vi "Teleop.vi"(10 "Match Info":T1={"Autonomous Elapsed Seconds"=0.0, "TeleOp Elapsed Seconds"=0.0, "Disabled Elapsed Seconds"=0.0, "Visited Autonomous"=FALSE, "Visited TeleOp"=FALSE, "Visited Disabled"=FALSE, "Autonomous Settings"={"Autonomous Style"=enum."Independent", "VI Refnum"=refnum}}, 11 "Call Context":T2) -> ()   [LabVIEW 2014]
doc: "This VI is called for each TeleOp packet received from the DS where the robot is not disabled. It is often used to read from the joysticks and update I/O or to update setpoints for timed control loops. It should complete and return within 20 milliseconds or it may miss DS packets."
uses:
  <vilib>/Rock Robotics/WPI/DriverStation/WPI_DriverStationDerivedRobotMode.ctl
  <vilib>/Rock Robotics/WPI/DriverStation/WPI_DriverStationMatch Info.ctl
  <vilib>/Rock Robotics/WPI/RobotDrive/WPI_RobotDriveGetSetRefNum.vi
  <vilib>/Rock Robotics/WPI/Joystick/WPI_JoystickGetSetRefNum.vi
  <vilib>/Rock Robotics/Network Tables/SD Write Boolean Array.vi
  <vilib>/Rock Robotics/Network Tables/SD Write Numeric Array.vi
  Robot Global Data.vi
  <vilib>/Rock Robotics/Network Tables/SD Read Boolean.vi
  <vilib>/Rock Robotics/Network Tables/SD Read Number.vi
panel:
  out "Sample Slider 0":dbl(slide) scale=0.0..5.0
  out "Sample Boolean 1":bool
  out "Sample Boolean 0":bool
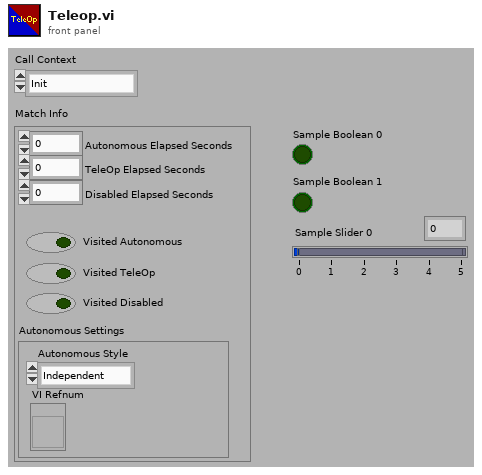
[diagram p1: front panel]
types:
  T1 = typedef "WPI_DriverStationMatch Info.ctl" = cluster{"Autonomous Elapsed Seconds":dbl, "TeleOp Elapsed Seconds":dbl, "Disabled Elapsed Seconds":dbl, "Visited Autonomous":bool, "Visited TeleOp":bool, "Visited Disabled":bool, "Autonomous Settings":cluster{"Autonomous Style":enum16{"Iterative", "Independent"}, "VI Refnum":refnum<vi>}}
  T2 = typedef "WPI_DriverStationDerivedRobotMode.ctl" = enum16{"Init", "Execute", "Stop"}
  T3 = typedef "WPI_RobotDriveDevRef.ctl" = cluster{"DevStatus":errorcluster, "Motors[]":T4[], "Square Inputs":bool, "Max Output":dbl}
  T4 = typedef "WPI_MotorControlDeviceRef.ctl" = cluster{"DeviceStatus":errorcluster, "Type":T5, "PWM":cluster{"Controller":T6, "PWM Channel":T7, "DeadBand":T8}, "CAN":cluster{"Device Number":u8, "Control Mode":T9, "Semaphore":T10, "Max Vout":dbl, "TalonSRX Control Mode":T11}, "Invert":bool, "TransformRef":T12, "InvTransformRef":T12}
  T5 = typedef "WPI_MotorControlType.ctl" = enum16{"PWM", "CAN", "CANTalonSRX"}
  T6 = typedef "FPGA_TypedefDigitalModule.ctl" = enum16{"Controller 1"}
  T7 = typedef "FPGA_DIOPWMChannel.ctl" = enum8{"PWM 0", "PWM 1", "PWM 2", "PWM 3", "PWM 4", "PWM 5", "PWM 6", "PWM 7", "PWM 8", "PWM 9", "PWM MXP 0", "PWM MXP 1", "PWM MXP 2", "PWM MXP 3", "PWM MXP 4", "PWM MXP 5", "PWM MXP 6", "PWM MXP 7", "PWM MXP 8", "PWM MXP 9", "Invalid"}
  T8 = typedef "WPI_PWMDeadband.ctl" = cluster{"Name":string, "maxPositivePwm":i32, "minPositivePwm":i32, "centerPwm":i32, "maxNegativePwm":i32, "minNegativePwm":i32, "angularRange":u16}
  T9 = typedef "WPI_CANJaguar_ControlMode.ctl" = enum8{"Percent VBus", "Current", "Speed", "Position", "Voltage"}
  T10 = typedef "Semaphore RefNum" = refnum<k1>
  T11 = typedef "WPI_CANTalonSRX_APIControlMode.ctl" = enum8{"Percent VBus", "Speed", "Position", "Slave", "Unchanged / Invalid"}
  T12 = typedef "WPI_PWMTransform_ConPane.ctl" = refnum<vi>
  T13 = typedef "WPI_JoystickDevRef.ctl" = cluster{"Device":T14}
  T14 = typedef "WPI_JoystickDeviceEnum.ctl" = enum16{"USB 0", "USB 1", "USB 2", "USB 3", "USB 4", "USB 5"}
  T15 = cluster{"Buttons[0]":bool, "Buttons[1]":bool, "Buttons[2]":bool, "Buttons[3]":bool, "Buttons[4]":bool, "Buttons[5]":bool, "Buttons[6]":bool, "Buttons[7]":bool, "Buttons[8]":bool}
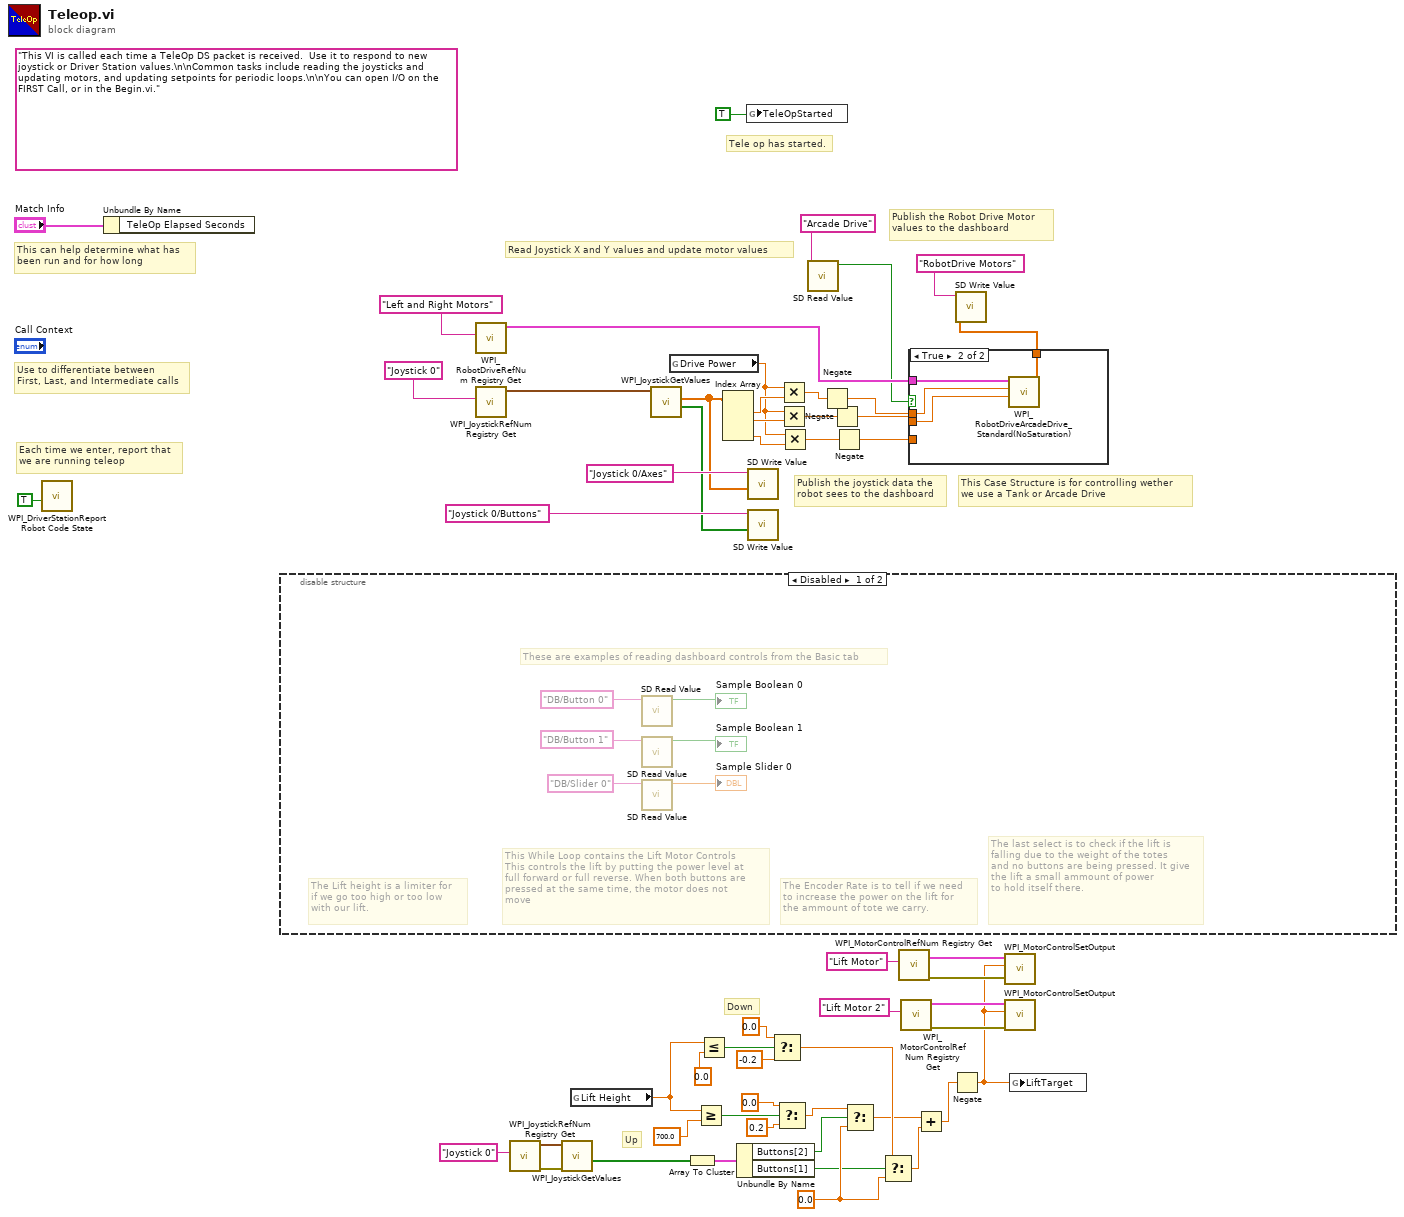
[diagram p0: block diagram]
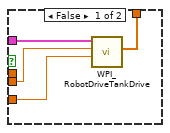
[diagram p3: hidden frame]
diagram:
  w20 = 0.0
  (unwired) "This VI is called each time a TeleOp DS packet is received.  Use it to respond to new joystick or Driver Station values.\n\nCommon tasks include reading the joysticks and updating motors, and updating setpoints for periodic loops.\n\nYou can open I/O on the FIRST Call, or in the Begin.vi."
  # "Read Joystick X and Y values and update motor values"
  # "Up"
  # "Down"
  # "Tele op has started."
  # "This Case Structure is for controlling wether\nwe use a Tank or Arcade Drive"
  # "Publish the Robot Drive Motor\nvalues to the dashboard"
  # "Publish the joystick data the\nrobot sees to the dashboard"
  # "Each time we enter, report that\nwe are running teleop"
  # "Use to differentiate between\nFirst, Last, and Intermediate calls"
  # "This can help determine what has\nbeen run and for how long"
  n1 = call <vilib>:"WPI_DriverStationReport Robot Code State.vi"("TeleOp"=TRUE ("Autonomous")) -> ()  [unwired: 10 in, 1 out]
  n2 = Unbundle By Name("Match Info") -> ()  [unwired: 1 out]
  n3 = disable-structure shown="Disabled" {
    frame Disabled {
      # "The last select is to check if the lift is falling due to the weight of the totes\nand no buttons are being pressed. It give the lift a small ammount of power\nto hold itself there."
      # "The Encoder Rate is to tell if we need\nto increase the power on the lift for\nthe ammount of tote we carry."
      # "The Lift height is a limiter for \nif we go too high or too low\nwith our lift."
      # "This While Loop contains the Lift Motor Controls\nThis controls the lift by putting the power level at\nfull forward or full reverse. When both buttons are\npressed at the same time, the motor does not\nmove"
      # "These are examples of reading dashboard controls from the Basic tab"
      n4 = call-poly <vilib>:"SD Read Value.vi"("Name"="DB/Button 0" ("refnum name")) -> ("Boolean"=→"Sample Boolean 0":bool)  [unwired: 8 in, 2 out]
      n5 = call-poly <vilib>:"SD Read Value.vi"("Name"="DB/Button 1" ("refnum name")) -> ("Boolean"=→"Sample Boolean 1":bool)  [unwired: 8 in, 2 out]
      n6 = call-poly <vilib>:"SD Read Value.vi"("Name"="DB/Slider 0" ("refnum name")) -> ("Numeric"=→"Sample Slider 0":dbl)  [unwired: 8 in, 2 out]
    }
    frame Enabled {
    }
  }
  n7 = call <vilib>:"WPI_RobotDriveRefNum Registry Get.vi"("refnum name"="Left and Right Motors") -> ("RobotDriveDevRef"=w38:T3)  [unwired: 1 in, 9 out]
  n8 = call <vilib>:"WPI_JoystickRefNum Registry Get.vi"("refnum name"="Joystick 0") -> ("JoystickDevRef"=w51:T13)  [unwired: 1 in, 9 out]
  n9 = call <vilib>:"WPI_JoystickRefNum Registry Get.vi"("refnum name"="Joystick 0") -> ("error out"=w29:errorcluster, "JoystickDevRef"=w30:T13)  [unwired: 9 in]
  n10 = call <vilib>:"WPI_JoystickGetValues.vi"("error in (no error)"=w29, "JoystickDevRef"=w30) -> ("Buttons"=w21:bool[])  [unwired: 5 in, 4 out]
  n11 = global read "Robot Global Data.vi" "Lift Height"() -> (w7:dbl)
  n12 = call <vilib>:"WPI_JoystickGetValues.vi"("JoystickDevRef"=w51) -> ("Buttons"=w45:bool[], "Axes"=w32:dbl[])  [unwired: 6 in, 3 out]
  n13 = global read "Robot Global Data.vi" "Drive Power"() -> (w39:dbl)
  n14 = Array To Cluster(array=w21) -> (cluster=w22:T15)
  n15 = Greater Or Equal?(x=w7, y=700.0) -> (x >= y?=w18:bool)
  n16 = Less Or Equal?(x=w7, y=0.0) -> (x <= y?=w14:bool)
  n17 = Index Array(array=w32) -> (element #1=w44:dbl, element #2=w41:dbl, element #4=w34:dbl)  [unwired: 4 in, 1 out]
  n18 = Unbundle By Name(w22) -> ("Buttons[2]"=w9:bool, "Buttons[1]"=w8:bool)
  n19 = global write "Robot Global Data.vi" "TeleOpStarted"(TRUE) -> ()
  n20 = call-poly <vilib>:"SD Write Value.vi"("Numeric Array"=w32, "Name"="Joystick 0/Axes") -> ()  [unwired: 8 in, 2 out]
  n21 = call-poly <vilib>:"SD Write Value.vi"("Boolean Array"=w45, "Name"="Joystick 0/Buttons") -> ()  [unwired: 8 in, 2 out]
  n22 = Select(t=0.0, s=w14, f=-0.2) -> (s? t:f=w12:dbl)
  n23 = Select(t=0.0, s=w18, f=0.2) -> (s? t:f=w17:dbl)
  n24 = Multiply(x=w39, y=w44) -> (x*y=w43:dbl)
  n25 = Multiply(x=w39, y=w41) -> (x*y=w40:dbl)
  n26 = Multiply(x=w39, y=w34) -> (x*y=w42:dbl)
  n27 = call-poly <vilib>:"SD Read Value.vi"("Name"="Arcade Drive") -> ("Boolean"=w1:bool)  [unwired: 8 in, 2 out]
  n28 = Negate(x=w43) -> (-x=w37:dbl)
  n29 = Negate(x=w40) -> (-x=w36:dbl)
  n30 = Negate(x=w42) -> (-x=w35:dbl)
  n31 = Select(t=w17, s=w9, f=w20) -> (s? t:f=w6:dbl)
  n32 = Select(t=w12, s=w8, f=w20) -> (s? t:f=w19:dbl)
  n33 = call <vilib>:"WPI_MotorControlRefNum Registry Get.vi"("refnum name"="Lift Motor") -> ("error out"=w25:errorcluster, "MotorControlDevRef"=w28:T4)  [unwired: 9 in]
  n34 = call <vilib>:"WPI_MotorControlRefNum Registry Get.vi"("refnum name"="Lift Motor 2") -> ("error out"=w26:errorcluster, "MotorControlDevRef"=w27:T4)  [unwired: 9 in]
  n35 = case shown="True" w1 {
    tunnel: w38 -> [w64 w68]
    tunnel: w37 -> [_ w67]
    tunnel: w36 -> [w61 w66]
    tunnel: [w63 w65] -> w48
    tunnel: w35 -> [w62 _]
    frame False {
      n36 = call <vilib>:"WPI_RobotDriveTankDrive.vi"("Right axis value"=w62, "Left axis value"=w61, "RobotDriveDevRef"=w64) -> ("Motor Values"=w63:dbl[])  [unwired: 6 in, 2 out]
    }
    frame True {
      n37 = call <vilib>:"WPI_RobotDriveArcadeDrive_Standard(NoSaturation).vi"("Y axis value"=w66, "X axis value"=w67, "RobotDriveDevRef"=w68) -> ("Motor Values"=w65:dbl[])  [unwired: 1 in, 7 out]
    }
  }
  n38 = Add(x=w6, y=w19) -> (x+y=w4:dbl)
  n39 = Negate(x=w4) -> (-x=w3:dbl)
  n40 = call-poly <vilib>:"SD Write Value.vi"("Numeric Array"=w48, "Name"="RobotDrive Motors") -> ()  [unwired: 8 in, 2 out]
  n41 = call <vilib>:"WPI_MotorControlSetOutput.vi"("error in (no error)"=w25, "Output"=w3, "MotorControlDevRef"=w28) -> ()  [unwired: 6 in, 3 out]
  n42 = call <vilib>:"WPI_MotorControlSetOutput.vi"("error in (no error)"=w26, "Output"=w3, "MotorControlDevRef"=w27) -> ()  [unwired: 6 in, 3 out]
  n43 = global write "Robot Global Data.vi" "LiftTarget"(w3) -> ()
